vi "MFC_read.vi"() -> ()   [LabVIEW 2013]
uses:
  GlobalStop.vi
  GlobalMFCread.vi
panel:
  out "error out 5":errorcluster
  out "error out 4":errorcluster
  out "error out 3":errorcluster
  out "error out 2":errorcluster
  out "error out":errorcluster
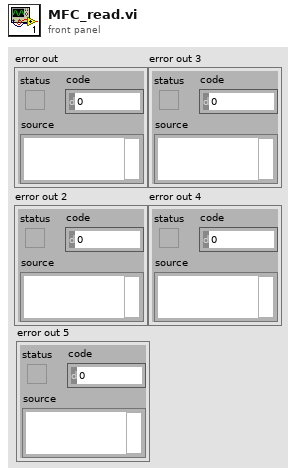
[diagram p1: front panel]
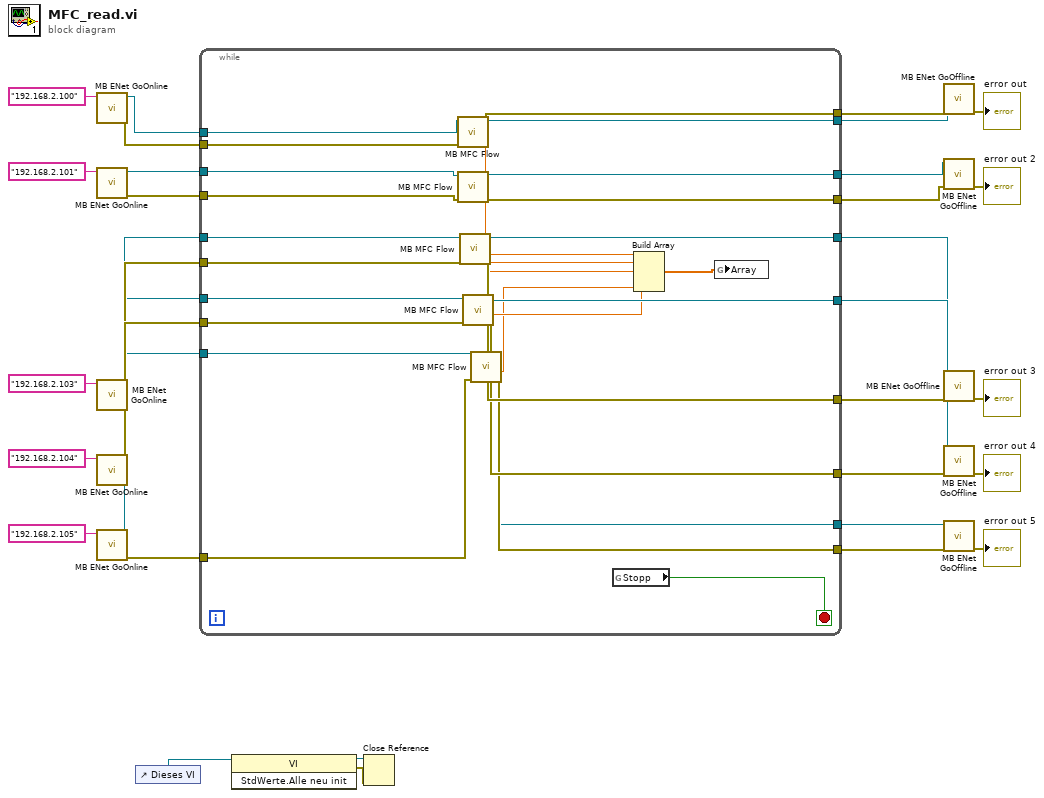
[diagram p0: block diagram]
diagram:
  n1 = call "MB ENet GoOnline.vi"("IP Address"="192.168.2.100") -> ("error out"=w19:errorcluster, "TCP Ref"=w8:refnum<k5>)  [unwired: 8 in, 1 out]
  n2 = call "MB ENet GoOnline.vi"("IP Address"="192.168.2.101") -> ("error out"=w20:errorcluster, "TCP Ref"=w7:refnum<k5>)  [unwired: 8 in, 1 out]
  n3 = call "MB ENet GoOnline.vi"("IP Address"="192.168.2.103") -> ("error out"=w21:errorcluster, "TCP Ref"=w6:refnum<k5>)  [unwired: 8 in, 1 out]
  n4 = call "MB ENet GoOnline.vi"("IP Address"="192.168.2.104") -> ("error out"=w22:errorcluster, "TCP Ref"=w5:refnum<k5>)  [unwired: 8 in, 1 out]
  n5 = call "MB ENet GoOnline.vi"("IP Address"="192.168.2.105") -> ("error out"=w23:errorcluster, "TCP Ref"=w4:refnum<k5>)  [unwired: 8 in, 1 out]
  n6 = control-ref of="Dieses VI"() -> (w3:refnum<vi>)
  n7 = while {
    tunnel: w23 -> [w60]
    tunnel: w22 -> [w59]
    tunnel: w21 -> [w58]
    tunnel: w20 -> [w57]
    tunnel: w19 -> [w56]
    tunnel: [w55] -> w18
    tunnel: [w54] -> w17
    tunnel: [w53] -> w16
    tunnel: [w52] -> w15
    tunnel: [w51] -> w14
    tunnel: [w50] -> w13
    tunnel: [w49] -> w12
    tunnel: [w48] -> w11
    tunnel: [w47] -> w10
    tunnel: [w46] -> w9
    tunnel: w8 -> [w45]
    tunnel: w7 -> [w44]
    tunnel: w6 -> [w43]
    tunnel: w5 -> [w42]
    tunnel: w4 -> [w41]
    stop <- w34 stop-if-true
    n8 = call "MB MFC Flow.vi"("error in (no error)"=w56, "TCP Ref"=w45) -> ("error out"=w55:errorcluster, "Flow(sccm)"=w40:sgl, "dup TCP Ref"=w46:refnum<k5>)  [unwired: 7 in]
    n9 = call "MB MFC Flow.vi"("error in (no error)"=w57, "TCP Ref"=w44) -> ("error out"=w54:errorcluster, "Flow(sccm)"=w39:sgl, "dup TCP Ref"=w47:refnum<k5>)  [unwired: 7 in]
    n10 = call "MB MFC Flow.vi"("error in (no error)"=w58, "TCP Ref"=w43) -> ("error out"=w53:errorcluster, "Flow(sccm)"=w38:sgl, "dup TCP Ref"=w48:refnum<k5>)  [unwired: 7 in]
    n11 = call "MB MFC Flow.vi"("error in (no error)"=w59, "TCP Ref"=w42) -> ("error out"=w52:errorcluster, "Flow(sccm)"=w37:sgl, "dup TCP Ref"=w49:refnum<k5>)  [unwired: 7 in]
    n12 = call "MB MFC Flow.vi"("error in (no error)"=w60, "TCP Ref"=w41) -> ("error out"=w51:errorcluster, "Flow(sccm)"=w36:sgl, "dup TCP Ref"=w50:refnum<k5>)  [unwired: 7 in]
    n13 = global read "GlobalStop.vi" "Stopp"() -> (w34:bool)
    n14 = Build Array(w40, w39, w38, w37, w36) -> (w35:sgl[])
    n15 = global write "GlobalMFCread.vi" "Array"(w35) -> ()
  }
  n16 = invoke class="VI" method="StdWerte.Alle neu init"(reference=w3) -> (reference out=w2:refnum<vi>, error out=w1:errorcluster)  [unwired: 2 in, 1 out]
  n17 = Close Reference(reference=w2, error in (no error)=w1) -> ()  [unwired: 1 out]
  n18 = call "MB ENet GoOffline.vi"("error in (no error)"=w18, "TCP Ref:ValBlock"=w9) -> ("error out"=→"error out":errorcluster)  [unwired: 7 in, 2 out]
  n19 = call "MB ENet GoOffline.vi"("error in (no error)"=w17, "TCP Ref:ValBlock"=w10) -> ("error out"=→"error out 2":errorcluster)  [unwired: 7 in, 2 out]
  n20 = call "MB ENet GoOffline.vi"("error in (no error)"=w16, "TCP Ref:ValBlock"=w11) -> ("error out"=→"error out 3":errorcluster)  [unwired: 7 in, 2 out]
  n21 = call "MB ENet GoOffline.vi"("error in (no error)"=w15, "TCP Ref:ValBlock"=w12) -> ("error out"=→"error out 4":errorcluster)  [unwired: 7 in, 2 out]
  n22 = call "MB ENet GoOffline.vi"("error in (no error)"=w14, "TCP Ref:ValBlock"=w13) -> ("error out"=→"error out 5":errorcluster)  [unwired: 7 in, 2 out]
